vi "SeqMgr.Compare String-Number Values.vi"(9 "Input 2":string, 10 "Input 1":string, 11 "Comparison":string) -> (0 "error":errorcluster, 1 "Are Numbers":bool, 3 "T/F":bool)   [LabVIEW 2024, in "EQMF.lvlib" / "SeqMgr.lvlib"]
uses:
  SeqMgr.lvlib
  <vilib>/Utility/error.llb/Trim Whitespace One-Sided.vi
panel:
  out "Num2":bool
  out "Num1":bool
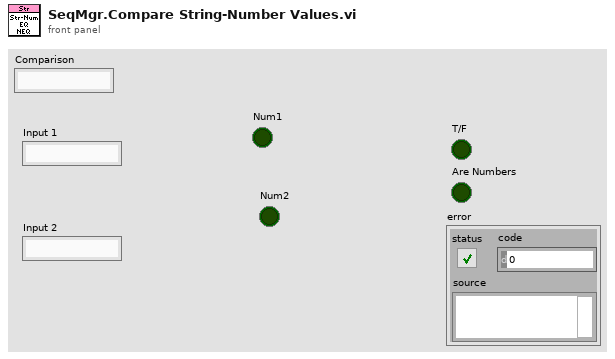
[diagram p1: front panel]
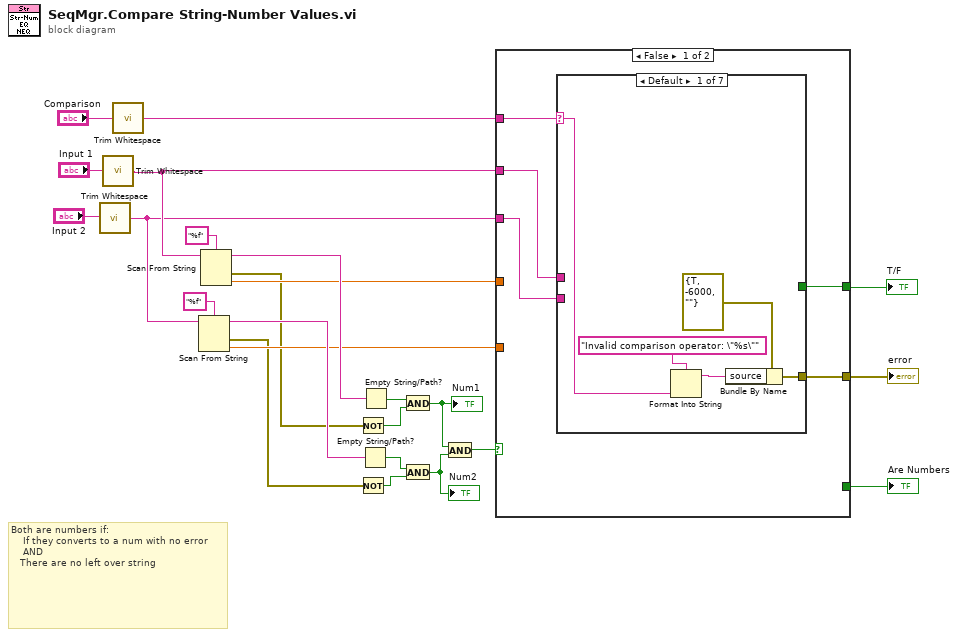
[diagram p0: block diagram]
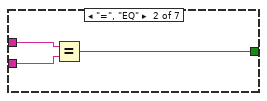
[diagram p2: hidden frame]
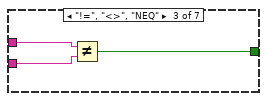
[diagram p3: hidden frame]
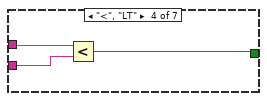
[diagram p4: hidden frame]
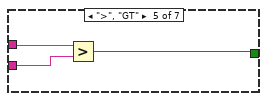
[diagram p5: hidden frame]
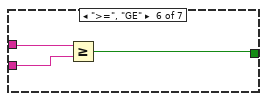
[diagram p6: hidden frame]
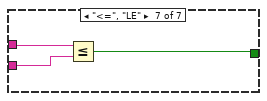
[diagram p7: hidden frame]
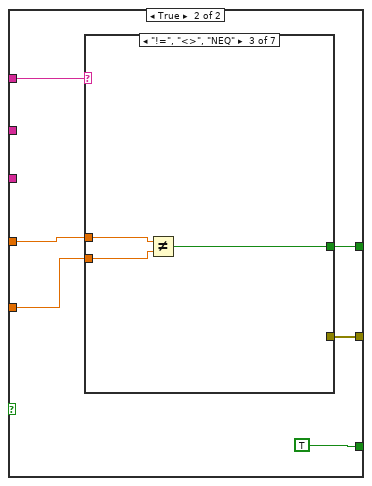
[diagram p8: hidden frame]
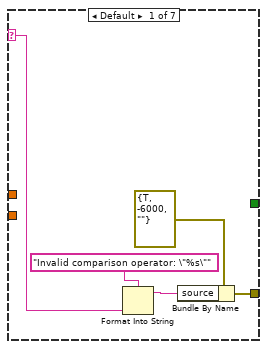
[diagram p9: hidden frame]
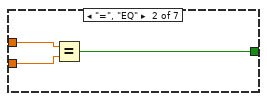
[diagram p10: hidden frame]
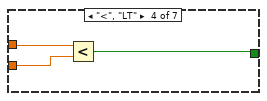
[diagram p11: hidden frame]
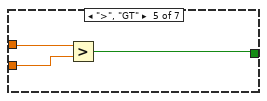
[diagram p12: hidden frame]
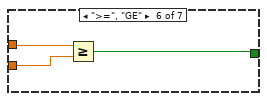
[diagram p13: hidden frame]
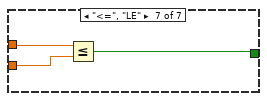
[diagram p14: hidden frame]
diagram:
  # "Both are numbers if:\n    If they converts to a num with no error\n    AND\n   There are no left over string"
  n1 = call <vilib>:"Trim Whitespace.vi"("string"="Input 2") -> ("trimmed string"=w14:string)  [unwired: 1 in]
  n2 = call <vilib>:"Trim Whitespace.vi"("string"="Input 1") -> ("trimmed string"=w16:string)  [unwired: 1 in]
  n3 = call <vilib>:"Trim Whitespace.vi"("string"="Comparison") -> ("trimmed string"=w1:string)  [unwired: 1 in]
  n4 = Scan From String(format string="%f", input string=w14) -> (remaining string=w22:string, error out=w6:errorcluster, output 1=w19:dbl)  [unwired: 3 in, 1 out]
  n5 = Scan From String(format string="%f", input string=w16) -> (remaining string=w23:string, error out=w9:errorcluster, output 1=w20:dbl)  [unwired: 3 in, 1 out]
  n6 = Not(x=w9) -> (.not. x?=w11:bool)
  n7 = Not(x=w6) -> (.not. x?=w8:bool)
  n8 = Empty String/Path?(string/path=w22) -> (empty?=w7:bool)
  n9 = Empty String/Path?(string/path=w23) -> (empty?=w10:bool)
  n10 = And(x=w10, y=w11) -> (x .and. y?=w4:bool)
  "Num1" <- w4
  n11 = And(x=w7, y=w8) -> (x .and. y?=w5:bool)
  "Num2" <- w5
  n12 = And(x=w4, y=w5) -> (x .and. y?=w18:bool)
  n13 = case shown="False" w18 {
    tunnel: w20 -> [_ w55]
    tunnel: w19 -> [_ w54]
    tunnel: w16 -> [w28 _]
    tunnel: w14 -> [w27 _]
    tunnel: [w26 w56] -> w13
    tunnel: [_ TRUE] -> w12
    tunnel: w1 -> [w29 w53]
    tunnel: [w25 w57] -> w3
    frame False {
      n14 = case shown="Default" w29 {
        selector: w29 -> [w30 _ _ _ _ _ _]
        tunnel: [w33 _ _ _ _ _ _] -> w25
        tunnel: w28 -> [_ w37 w40 w43 w46 w49 w52]
        tunnel: w27 -> [_ w36 w39 w42 w45 w48 w51]
        tunnel: [_ w35 w38 w41 w44 w47 w50] -> w26
        frame Default {
          n15 = Format Into String(format string="Invalid comparison operator: \"%s\"" ("source"), w30) -> (resulting string=w31:string)  [unwired: 2 in, 1 out]
          n16 = Bundle By Name(cluster=errorcluster {"status"=TRUE, "code"=-6000, "source"=""} ("error constant"), "source"=w31) -> (w33:errorcluster)
        }
        frame "=", "EQ" {
          n17 = Equal?(x=w37, y=w36) -> (x = y?=w35:bool)
        }
        frame "!=", "<>", "NEQ" {
          n18 = Not Equal?(x=w40, y=w39) -> (x != y?=w38:bool)
        }
        frame "<", "LT" {
          n19 = Less?(x=w43, y=w42) -> (x < y?=w41:bool)
        }
        frame ">", "GT" {
          n20 = Greater?(x=w46, y=w45) -> (0:w44:bool)
        }
        frame ">=", "GE" {
          n21 = Greater Or Equal?(x=w49, y=w48) -> (x >= y?=w47:bool)
        }
        frame "<=", "LE" {
          n22 = Less Or Equal?(x=w52, y=w51) -> (x <= y?=w50:bool)
        }
      }
    }
    frame True {
      n23 = case shown="\"!=\", \"<>\", \"NEQ\"" w53 {
        selector: w53 -> [w59 _ _ _ _ _ _]
        tunnel: [w62 _ _ _ _ _ _] -> w57
        tunnel: w55 -> [_ w66 w69 w72 w75 w78 w81]
        tunnel: w54 -> [_ w65 w68 w71 w74 w77 w80]
        tunnel: [_ w64 w67 w70 w73 w76 w79] -> w56
        frame Default {
          n24 = Format Into String(format string="Invalid comparison operator: \"%s\"" ("source"), w59) -> (resulting string=w60:string)  [unwired: 2 in, 1 out]
          n25 = Bundle By Name(cluster=errorcluster {"status"=TRUE, "code"=-6000, "source"=""} ("error constant"), "source"=w60) -> (w62:errorcluster)
        }
        frame "=", "EQ" {
          n26 = Equal?(x=w66, y=w65) -> (x = y?=w64:bool)
        }
        frame "!=", "<>", "NEQ" {
          n27 = Not Equal?(x=w69, y=w68) -> (x != y?=w67:bool)
        }
        frame "<", "LT" {
          n28 = Less?(x=w72, y=w71) -> (x < y?=w70:bool)
        }
        frame ">", "GT" {
          n29 = Greater?(x=w75, y=w74) -> (0:w73:bool)
        }
        frame ">=", "GE" {
          n30 = Greater Or Equal?(x=w78, y=w77) -> (x >= y?=w76:bool)
        }
        frame "<=", "LE" {
          n31 = Less Or Equal?(x=w81, y=w80) -> (x <= y?=w79:bool)
        }
      }
    }
  }
  "Are Numbers" <- w12
  "T/F" <- w13
  "error" <- w3
